vi "3.4.vi"() -> ()   [LabVIEW 2017]
panel:
  out "长度":i32
  out "连接后的字符串":string
  in  "数值":dbl
  in  "头":string
  in  "尾":string
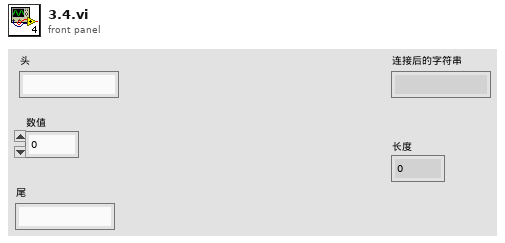
[diagram p1: front panel]
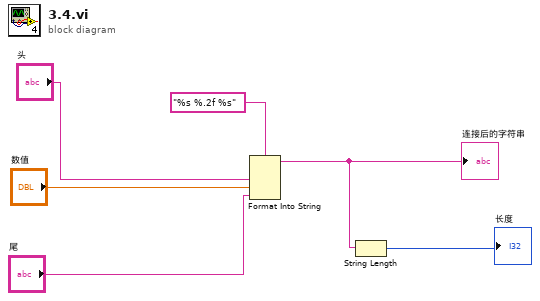
[diagram p0: block diagram]
diagram:
  n1 = Format Into String(format string="%s %.2f %s" ("格式字符串"), "头", "数值", "尾") -> (resulting string=w2:string)  [unwired: 2 in, 1 out]
  "连接后的字符串" <- w2
  n2 = String Length(string=w2) -> (length=→"长度":i32)
